vi "Write Timeout (ms).vi"(8 "error in (no error)":errorcluster, 10 "Timeout (ms)":i32, 11 "Wait On Integer Step in":refnum<class "Wait On Integer.lvclass">) -> (0 "error out":errorcluster, 3 "Wait On Integer Step out":refnum<class "Wait On Integer.lvclass">)   [LabVIEW 2015, in "Wait On Integer.lvclass"]
uses:
  Wait On Integer.lvclass
  Wait On Integer.lvclass/Wait On Integer.ctl
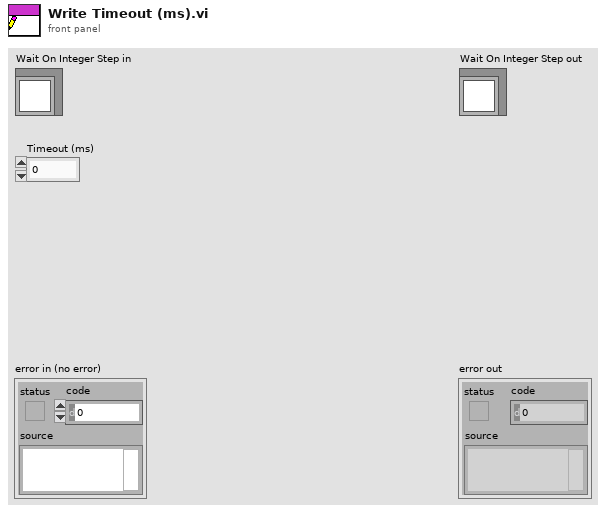
[diagram p1: front panel]
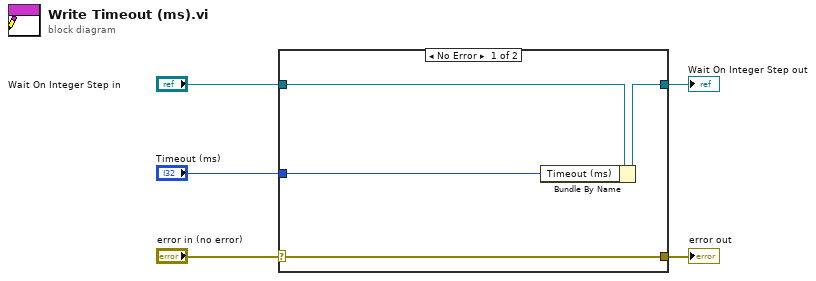
[diagram p0: block diagram]
diagram:
  n1 = case shown="No Error" "error in (no error)" {
    selector: "error in (no error)" -> [w9 w10]
    tunnel: [w9 w10] -> w4
    tunnel: [w7 w11] -> w2
    tunnel: "Wait On Integer Step in" -> [w8 w11]
    tunnel: "Timeout (ms)" -> [w6 _]
    frame No Error {
      n2 = Bundle By Name(cluster=w8, "Timeout (ms)"=w6) -> (w7:refnum<class "Wait On Integer.lvclass">)
    }
    frame Error {
    }
  }
  "error out" <- w4
  "Wait On Integer Step out" <- w2
